vi "Filter Cluster Items.vi"(7 "Action":T1, 10 "Filter Str":string, 11 "Display Items":T2[](array[typedef])) -> (3 "Filtered Items":T2[](array[typedef]))   [LabVIEW 2023]
uses:
  cluster/Cluster Element Description.ctl
  controls/action enum.ctl
  6f3da2d7-fab3-4264-b55d-857bcada8f4e.vi
  <userlib>/_OpenG.lib/array/array.llb/Filter 1D Array with Scalar (I32)__ogtk.vi
  <userlib>/_OpenG.lib/array/array.llb/Index 1D Array Elements (Variant)__ogtk.vi
panel:
  out "Array":cluster{"Array":string[]}[](array[cluster])
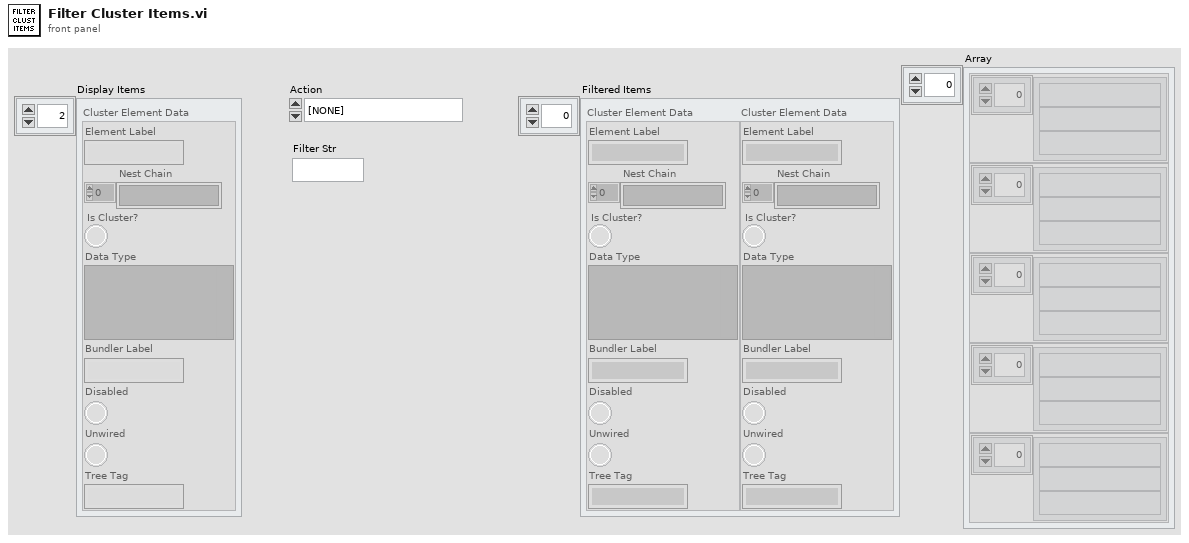
[diagram p1: front panel]
types:
  T1 = typedef "action enum.ctl" = enum16{"[NONE]", "Wire Bundle", "Wire Unbundle", "Terminal Unbundle", "Terminal Bundle", "Bundler Move Up", "Bundler Move Down", "Bundler Insert", "Bundler Remove", "Bundler Remove Unwired", "Bundler Rearrange", "In Place Insert", "In Place Remove", "In Place Remove Unwired", "In Place Rearrange", "Wire Properties", "Wire Method", "Terminal Properties", "Terminal Method", "Property Move Up", "Property Move Down", "Properties Insert", "Properties Remove", "Properties Remove Unwired", "Properties Rearrange", "Method Change", "Class for Constant", "Class For Control", "Class For Node", "Class Name to Clipboard"}
  T2 = typedef "Cluster Element Description.ctl" = cluster{"Element Label":string, "Nest Chain":string[], "Is Cluster?":bool, "Data Type":variant, "Bundler Label":string, "Disabled":bool, "Unwired":bool, "Tree Tag":string}
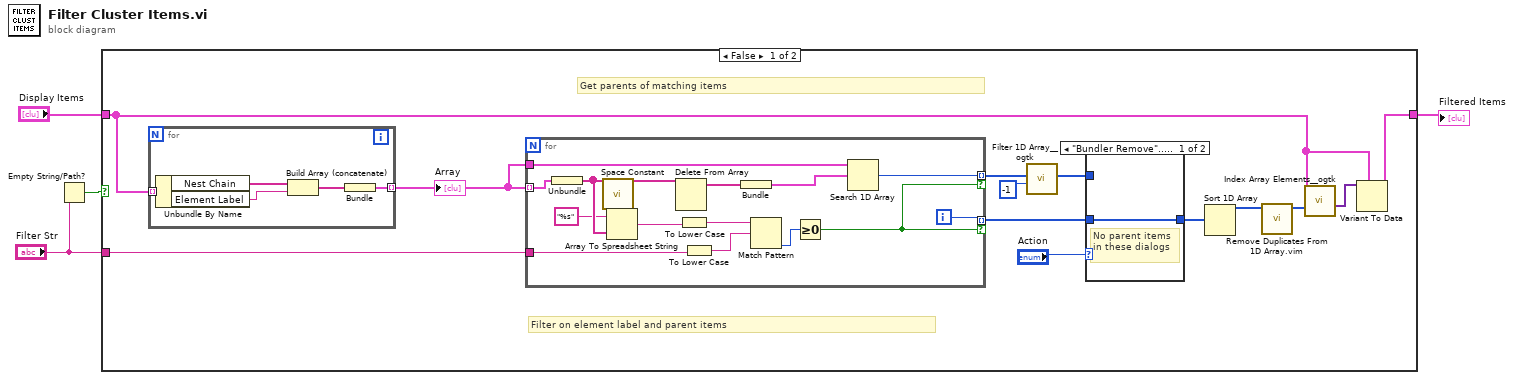
[diagram p0: block diagram]
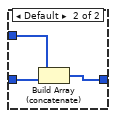
[diagram p2: hidden frame]
diagram:
  n1 = Empty String/Path?(string/path="Filter Str") -> (empty?=w1:bool)
  n2 = case shown="False" w1 {
    tunnel: [w6 w42] -> w4
    tunnel: "Display Items" -> [w5 w42]
    tunnel: "Filter Str" -> [w13 _]
    frame False {
      # "Filter on element label and parent items"
      # "Get parents of matching items"
      n3 = for {
        tunnel: w5 -> [w22] mode=indexing
        tunnel: [w18] -> w17 mode=indexing
        n4 = Unbundle By Name(w22) -> ("Nest Chain"=w21:string[], "Element Label"=w20:string)
        n5 = Build Array (concatenate)(w21, w20) -> (w19:string[])
        n6 = Bundle(w19) -> (w18:cluster{string[]})  [unwired: 1 in]
      }
      "Array" <- w17
      n7 = for {
        tunnel: w17 -> [w31] mode=indexing
        tunnel: w17 -> [w39]
        tunnel: [w40] -> w16 mode=indexing if=w35
        tunnel: [w36] -> w12 mode=indexing if=w35
        tunnel: w13 -> [w32]
        i -> [w40]
        n8 = Unbundle(w31) -> (w30:string[])
        n9 = call <vilib>:"Space Constant.vi"() -> ("String"=w28:string)
        n10 = Array To Spreadsheet String(delimiter (Tab)=w28, array=w30, 3:"%s" ("format string")) -> (spreadsheet string=w27:string)
        n11 = Delete From Array(array=w30) -> (array with subset deleted=w38:string[])  [unwired: 2 in, 1 out]
        n12 = To Lower Case(string=w27) -> (all lower case string=w34:string)
        n13 = To Lower Case(string=w32) -> (all lower case string=w33:string)
        n14 = Bundle(w38) -> (w37:cluster{string[]})  [unwired: 1 in]
        n15 = Match Pattern(string=w34, regular expression=w33) -> (offset past match=w41:i32)  [unwired: 1 in, 3 out]
        n16 = Greater Or Equal To 0?(x=w41) -> (x >= 0?=w35:bool)
        n17 = Search 1D Array(1D array=w39, element=w37) -> (index of element=w36:i32)  [unwired: 1 in]
      }
      n18 = call-poly <userlib>:"Filter 1D Array__ogtk.vi"("items to filter"=-1, "array"=w12) -> ("filtered array"=w10:i32[])  [unwired: 4 in, 1 out]
      n19 = case shown="\"Bundler Remove\"..\"Bundler Rearrange\"" "Action" {
        tunnel: w16 -> [w23 w26]
        tunnel: [w23 w25] -> w15
        tunnel: w10 -> [_ w24]
        frame "Bundler Remove".."Bundler Rearrange" {
          # "No parent items in these dialogs"
        }
        frame Default {
          n20 = Build Array (concatenate)(w24, w26) -> (w25:i32[])
        }
      }
      n21 = Sort 1D Array(array=w15) -> (sorted array=w14:i32[])
      n22 = call "Remove Duplicates From 1D Array.vim"("array"=w14) -> ("array with duplicates removed"=w8:i32[])  [unwired: 10 in]
      n23 = call-poly <userlib>:"Index Array Elements__ogtk.vi"("indices"=w8, "array"=w5) -> ("elements"=w7:variant[])  [unwired: 9 in]
      n24 = Variant To Data(type=w5, Variant=w7) -> (data=w6:T2[])  [unwired: 1 in, 1 out]
    }
    frame True {
    }
  }
  "Filtered Items" <- w4
